vi "Abort Sample Transfer.vi"(8 "error in (no error)":errorcluster, 11 "cRIO-CO2 in":refnum<class "cRIO-CO2.lvclass">) -> (0 "error out":errorcluster, 3 "cRIO-CO2 out":refnum<class "cRIO-CO2.lvclass">)   [LabVIEW 2015, in "cRIO-Carbondioxide.lvlib" / "cRIO-CO2.lvlib" / "cRIO-CO2.lvclass"]
uses:
  cRIO-CO2.lvclass
  Controls/Sample Transfer State Enumerator.ctl
  cRIO-CO2.lvclass/cRIO-CO2.ctl
  Send Time-delayed Transfer Sample.vi
  State Elapsed Time.vi
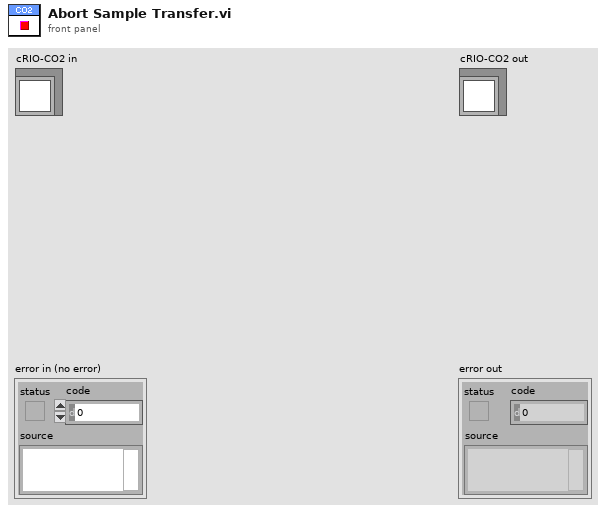
[diagram p1: front panel]
types:
  T1 = typedef "Sample Transfer State Enumerator.ctl" = enum16{"Idle", "Initialize", "Check Containers", "Check Temperatures", "Start Turbo", "Warm Up Containers", "Prepare for purging", "Purge Capillary", "Purge", "Open Containers", "Introduce Sample", "Measure Base Pressure", "Home Syringe", "Start Freezer", "Freeze Target", "Crystalize", "Initiate Stash", "Stash", "Polish", "Stop Freezers", "Push Sample", "Complete", "Abort", "Error", "Undefined"}
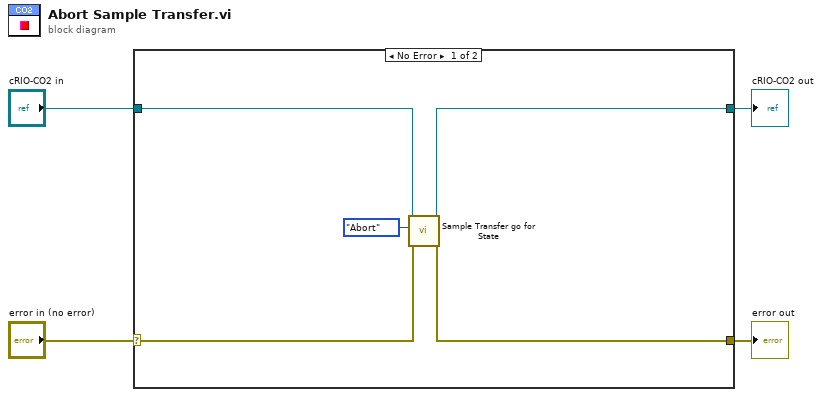
[diagram p0: block diagram]
diagram:
  n1 = case shown="No Error" "error in (no error)" {
    selector: "error in (no error)" -> [w7 w11]
    tunnel: [w6 w11] -> w3
    tunnel: [w8 w10] -> w1
    tunnel: "cRIO-CO2 in" -> [w9 w10]
    frame No Error {
      n2 = call "Sample Transfer go for State.vi"("error in (no error)"=w7, "Sample Transfer State"=Sample_Transfer_State_Enumerator."Abort", "cRIO-CO2 in"=w9) -> ("error out"=w6:errorcluster, "cRIO-CO2 out"=w8:refnum<class "cRIO-CO2.lvclass">)  [unwired: 7 in]
    }
    frame Error {
    }
  }
  "error out" <- w3
  "cRIO-CO2 out" <- w1
